vi "DAQmx Test.vi"   [LabVIEW 2023, in "VolatusScratch.lvlib"]
uses:
  VolatusScratch.lvlib
  Volatus/Volatus Core/Volatus Core.lvclass
  VolatusDAQ/VolatusDAQ.lvlib
  VolatusDAQGenericGUI/VolatusDAQGenericGUI.lvlib
  VolatusData/VolatusData.lvlib
panel:
  # "DAQmx Test App"
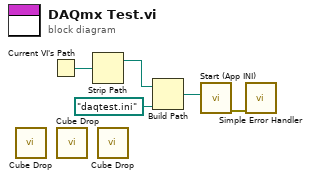
[diagram p0: block diagram]
diagram:
  n1 = call "Cube Drop.vi"() -> ()  [unwired: 12 in]
  n2 = Current VI's Path() -> (path=w2:path)
  n3 = call "Cube Drop.vi"() -> ()  [unwired: 12 in]
  n4 = Strip Path(path=w2) -> (stripped path=w1:path)  [unwired: 1 out]
  n5 = call "Cube Drop.vi"() -> ()  [unwired: 12 in]
  n6 = Build Path(base path=w1, name or relative path=path "daqtest.ini") -> (appended path=w3:path)
  n7 = call "Start (App INI).vi"("INI Path (Default)"=w3) -> ("error out"=w5:errorcluster)  [unwired: 9 in, 1 out]
  n8 = call <vilib>:"Simple Error Handler.vi"("error in (no error)"=w5) -> ()  [unwired: 4 in, 5 out]
